vi "Restart.LoadSettings.vi"(8 "error in":errorcluster, 11 "path (use dialog)":path) -> (0 "error out":errorcluster, 2 "Restart Settings":T1={"LogFile"=path "", "Log Settings"=[], "StimulusProfile"=path "", "StopIteration"=0, "StopStep"=0, "Log Channels"=enum."Aliases", "Base File Name"="Log", "Enable Logging"=TRUE, "Profile"="", "StopDuration"=0.0, "Waveform Definition"=path "", "Number of Cycles"=0.0, "Cyclic Frequency"=0.0, "Work Order Number"="", "Operator Name"="", "Description"="", "Station.ID"="", "Sequence.Channels"=[], "Alarms"=[]} {"Alarms"."Delay" format="%.2f"; "Alarms"."Low Limit" format="%.2f"; "Alarms"."High Limit" format="%.2f"}, 3 "path":path)   [LabVIEW 2015, in "Single Station Execution.lvlib"]
uses:
  Single Station Execution.lvlib
  Types/Restart.Settings.ctl
  <vilib>/NI Veristand/Execution/DataLogging/TDMS Channel Group.ctl
  <vilib>/NI Veristand/Execution/DataLogging/TDMS Property.ctl
  <vilib>/NI Veristand/Execution/DataLogging/TDMS Channel.ctl
  <vilib>/NI Veristand/Execution/DataLogging/Time Channel Options.ctl
  Types/Log.SelectedChannels.ctl
  Types/Config.AlarmSettings.ctl
  Main.Constants.vi
  <vilib>/NI/GXML/_subVIs/GXML Quick Parser/Quick Parser.vi
  <vilib>/NI/GXML/GXML.lvlib
  <vilib>/NI Veristand/Execution/DataLogging/NI_VS Data Logging API.lvlib
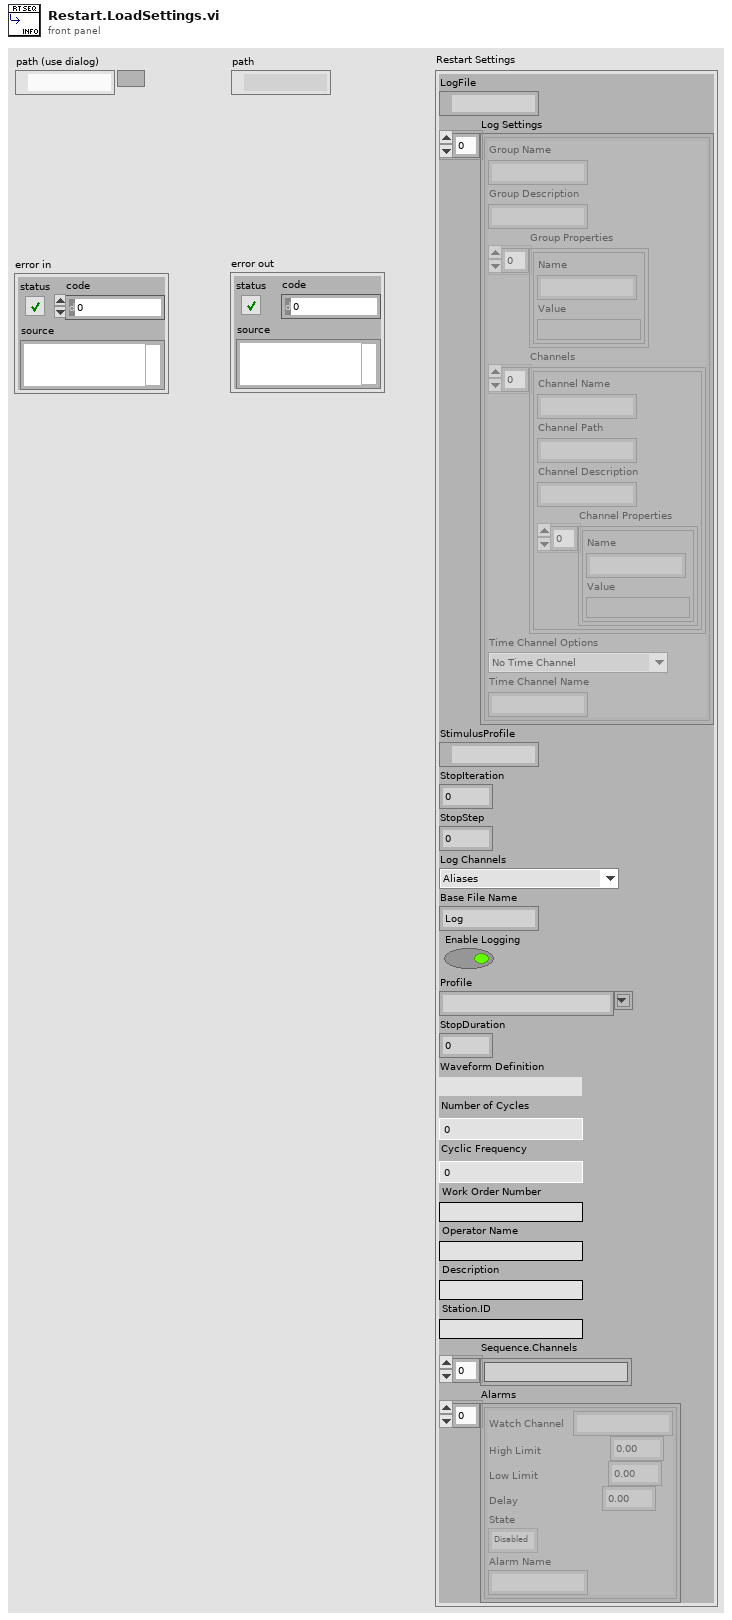
[diagram p1: front panel]
types:
  T1 = typedef "Single Station Execution.lvlib/Restart.Settings.ctl" = cluster{"LogFile":path, "Log Settings":T2[], "StimulusProfile":path, "StopIteration":u32, "StopStep":u32, "Log Channels":T6, "Base File Name":string, "Enable Logging":bool, "Profile":string, "StopDuration":dbl, "Waveform Definition":path, "Number of Cycles":dbl, "Cyclic Frequency":dbl, "Work Order Number":string, "Operator Name":string, "Description":string, "Station.ID":string, "Sequence.Channels":string[], "Alarms":T7[]}
  T2 = typedef "NI_VS Data Logging API.lvlib/TDMS Channel Group.ctl" = cluster{"Group Name":string, "Group Description":string, "Group Properties":T3[], "Channels":T4[], "Time Channel Options":T5, "Time Channel Name":string}
  T3 = typedef "NI_VS Data Logging API.lvlib/TDMS Property.ctl" = cluster{"Name":string, "Value":variant}
  T4 = typedef "NI_VS Data Logging API.lvlib/TDMS Channel.ctl" = cluster{"Channel Name":string, "Channel Path":string, "Channel Description":string, "Channel Properties":T3[]}
  T5 = typedef "NI_VS Data Logging API.lvlib/Time Channel Options.ctl" = enum16{"No Time Channel", "Absolute Time", "System Time", "System Time - Microseconds", "Absolute Time as Double", "Relative To First Start Trigger", "Relative To Session Start"}
  T6 = typedef "Single Station Execution.lvlib/Log.SelectedChannels.ctl" = enum16{"Channels (No System Channel)", "Aliases", "All"}
  T7 = typedef "Single Station Execution.lvlib/Config.AlarmSettings.ctl" = cluster{"Watch Channel":string, "High Limit":dbl, "Low Limit":dbl, "Delay":dbl, "State":enum16{"Disabled", "Enabled", "Tripped", "Delayed Trip", "Indicate"}, "Alarm Name":string}
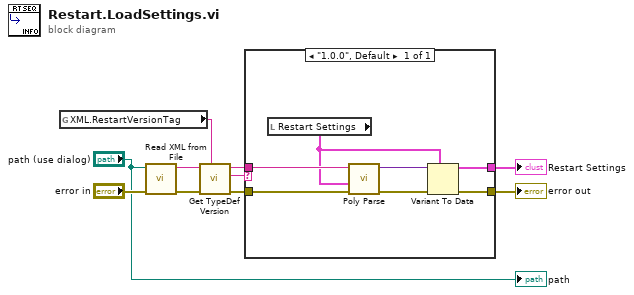
[diagram p0: block diagram]
diagram:
  n1 = global read "Main.Constants.vi" "XML.RestartVersionTag"() -> (w5:string)
  n2 = call <vilib>:"Read XML from File.vi"("error in"="error in", "XML File Path"="path (use dialog)") -> ("error out"=w10:errorcluster, "XML String Out"=w8:string)  [unwired: 8 in]
  n3 = call <vilib>:"Get TypeDef Version.vi"("Version Tag Name"=w5, "error in"=w10, "XML String In"=w8) -> ("error out"=w9:errorcluster, "Version String"=w6:string, "XML String Out"=w7:string)  [unwired: 6 in]
  n4 = case shown="\"1.0.0\", Default" w6 {
    tunnel: w9 -> [w15]
    tunnel: w7 -> [w14]
    tunnel: [w13] -> w4
    tunnel: [w12] -> w3
    frame "1.0.0", Default {
      n5 = local read "Restart Settings"() -> (w11:T1)
      n6 = call-poly <vilib>:"Poly Parse.vi"("error in"=w15, "TypeDesc"=w11, "XML File String"=w14) -> ("error out"=w17:errorcluster, "Parsed Data"=w16:variant)  [unwired: 7 in]
      n7 = Variant To Data(error in=w17, type=w11, Variant=w16) -> (data=w13:T1, error out=w12:errorcluster)
    }
  }
  "Restart Settings" <- w4
  "error out" <- w3
  "path" <- "path (use dialog)"
